vi "Test Websockets Requirements.vi"(8 "error in (no error)":errorcluster) -> (0 "error out":errorcluster)   [LabVIEW 2013]
uses:
  <vilib>/addons/_JKI Toolkits/Caraya/classes/Test/Test.lvclass
  source/Server class/Server.lvclass
  <vilib>/LabVIEW Open Source Project/MQTT Connection/MQTT_Base/Base Class/MQTT_Base.lvclass
  <vilib>/LabVIEW Open Source Project/Connection/Connection.Websockets/Connection.WS.lvclass
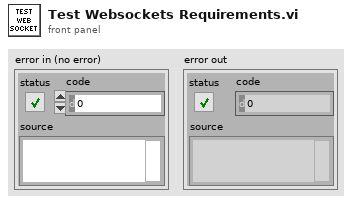
[diagram p1: front panel]
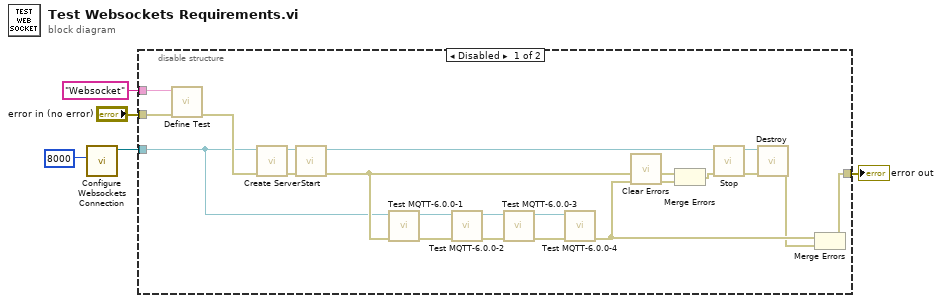
[diagram p0: block diagram]
diagram:
  n1 = call <vilib>:"Configure Websockets Connection.vi"("remote port (80)"=u16 8000) -> ("Connection.Websockets"=w1:refnum<class "Connection.WS.lvclass">)  [unwired: 9 in, 1 out]
  n2 = disable-structure shown="Disabled" {
    disable-tunnel: "Websocket" ("address (localhost)") -> [w26 _]
    disable-tunnel: "error in (no error)" -> [w18 w27]
    disable-tunnel: [w6 w27] -> w3
    disable-tunnel: w1 -> [w9 _]
    frame Disabled {
      n3 = call <vilib>:"Define Test.vi"("error in (no error)"=w18, "Label (VI Title)"=w26) -> ("error out"=w17:errorcluster)  [unwired: 9 in]
      n4 = call "Create Server.vi"("error in (no error)"=w17, "Connection Configuration"=w9) -> ("error out"=w24:errorcluster, "Server"=w25:refnum<class "Server.lvclass">)  [unwired: 8 in]
      n5 = call <vilib>:"Start.vi"("error in (no error)"=w24, "MQTT_Base in"=w25) -> ("error out"=w19:errorcluster, "MQTT_Base out"=w22:refnum<class "Server.lvclass">)  [unwired: 7 in, 1 out]
      n6 = call "Test MQTT-6.0.0-1.vi"("error in (no error)"=w19, "Connection"=w9) -> ("error out"=w7:errorcluster, "Connection"=w8:refnum<class "Connection.WS.lvclass">)  [unwired: 8 in]
      n7 = call "Test MQTT-6.0.0-2.vi"("error in (no error)"=w7, "Connection"=w8) -> ("error out"=w10:errorcluster, "Connection"=w11:refnum<class "Connection.WS.lvclass">)  [unwired: 8 in]
      n8 = call "Test MQTT-6.0.0-3.vi"("error in (no error)"=w10, "Connection"=w11) -> ("error out"=w12:errorcluster, "Connection"=w13:refnum<class "Connection.WS.lvclass">)  [unwired: 8 in]
      n9 = call "Test MQTT-6.0.0-4.vi"("error in (no error)"=w12, "Connection"=w13) -> ("error out"=w16:errorcluster)  [unwired: 8 in, 1 out]
      n10 = call <vilib>:"Clear Errors.vi"("error in (no error)"=w16) -> ("error out"=w14:errorcluster)  [unwired: 6 in]
      n11 = Merge Errors(w19, w14) -> (w21:errorcluster)
      n12 = call <vilib>:"Stop.vi"("error in (no error)"=w21, "MQTT_Base in"=w22) -> ("error out"=w20:errorcluster, "MQTT_Base out"=w23:refnum<class "Server.lvclass">)  [unwired: 7 in, 1 out]
      n13 = call <vilib>:"Destroy.vi"("error in (no error)"=w20, "MQTT_Base in"=w23) -> ("error out"=w15:errorcluster)  [unwired: 8 in, 1 out]
      n14 = Merge Errors(w16, w15) -> (w6:errorcluster)
    }
    frame Enabled {
    }
  }
  "error out" <- w3
